vi "Mindsensors Relay Driver Config.vi"(10 "Node Data":T3, 11 "NXT":T1) -> ()   [LabVIEW 2010]
uses:
  <vilib>/NXT/Subs/LVHSConnector.ctl
  Datatypes/Node.ctl
  UI Controls/PlugInControls/Pluginbackground.ctl
  <vilib>/NXT/Subs/MotorOutput.ctl
  <vilib>/Utility/miscctls.llb/LVPointTypeDef.ctl
  ConvertNodeAddrLEGOMotor.vi
  <vilib>/NXT/Dual Mode Library/Motors/MotorBrake.vi
  <vilib>/NXT/Dual Mode Library/Motors/MotorOn.vi
  <vilib>/NXT/Dual Mode Library/Motors/MotorReverse.vi
  <vilib>/NXT/Dual Mode Library/Motors/MotorCoast.vi
  ConvertNodeAddrSensor.vi
panel:
  in  "NXT 2":T1
  out "Output Port":T2=3 items=["Port A"=0, "Port B"=1, "Port C"=2, "Ports A & B"=4, "Ports A & C"=5, "Ports B & C"=6, "All Ports"=3]
  out "String":string
  in  "Relay":u16(ring) items=["Off", "Relay 1", "Relay 2"]
  in  "Device Address":string
  in  "NXT Port":string
  in  "Name":string
  out "Headline":string="Type (auto populated)"
  in  "Sensor Parameters":string
  in  "Instance Specific Data":cluster{"Example Data":dbl, "Numeric":dbl}
  in  "Reset":bool
  in  "Save":bool
  in  "Stop":bool
  out "Background":T4=TRUE
  # "<- No controls below this line"
  # "Common controls such as Buttons, Rings, Sliders, Graphs, Decorations, etc can be found in the <labview>\\Targets\\NI\\NXT\\NXT Toolkit\\Schematic Editor\\UI Controls\\Plugin Controls\\ folder. Use these controls when possible to ensure a consistent look and feel with LabVIEW Education Edition."
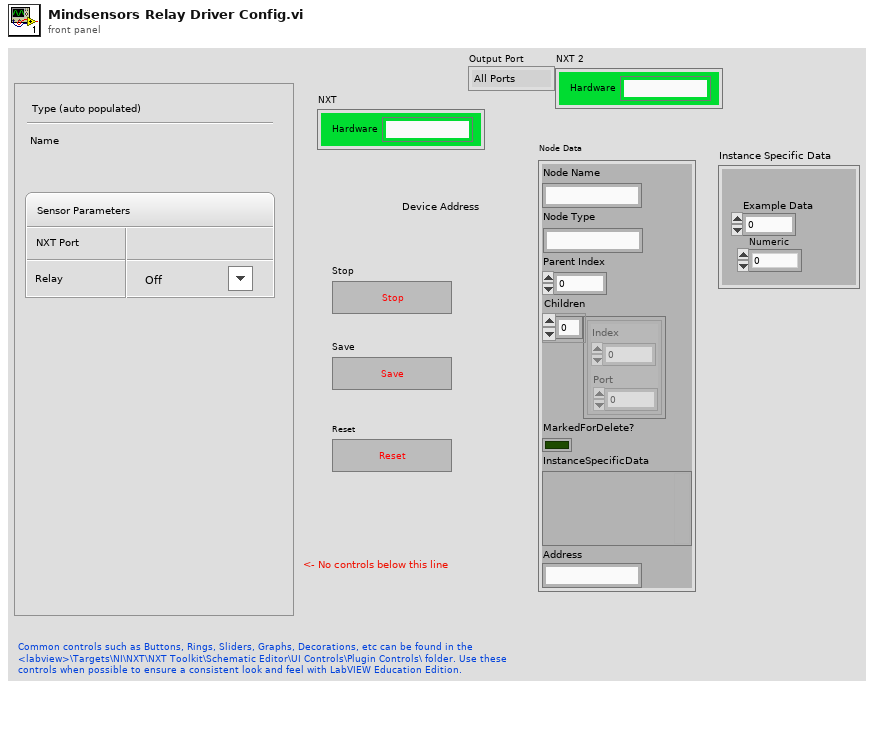
[diagram p1: front panel]
types:
  T1 = typedef "LVHSConnector.ctl" = cluster{"Hardware":string, "Flattened String":string}
  T2 = typedef "MotorOutput.ctl" = u8
  T3 = typedef "Node.ctl" = cluster{"Node Name":string, "Node Type":string, "Parent Index":i16, "Children":cluster{"Index":u16, "Port":u16}[], "MarkedForDelete?":bool, "InstanceSpecificData":variant, "Address":string}
  T4 = typedef "Pluginbackground.ctl" = bool
  T5 = typedef "LVPointTypeDef.ctl" = cluster{"Horizontal":i16, "Vertical":i16}
  T6 = enum8{"Enabled", "Disabled", "Disabled and Grayed Out"}
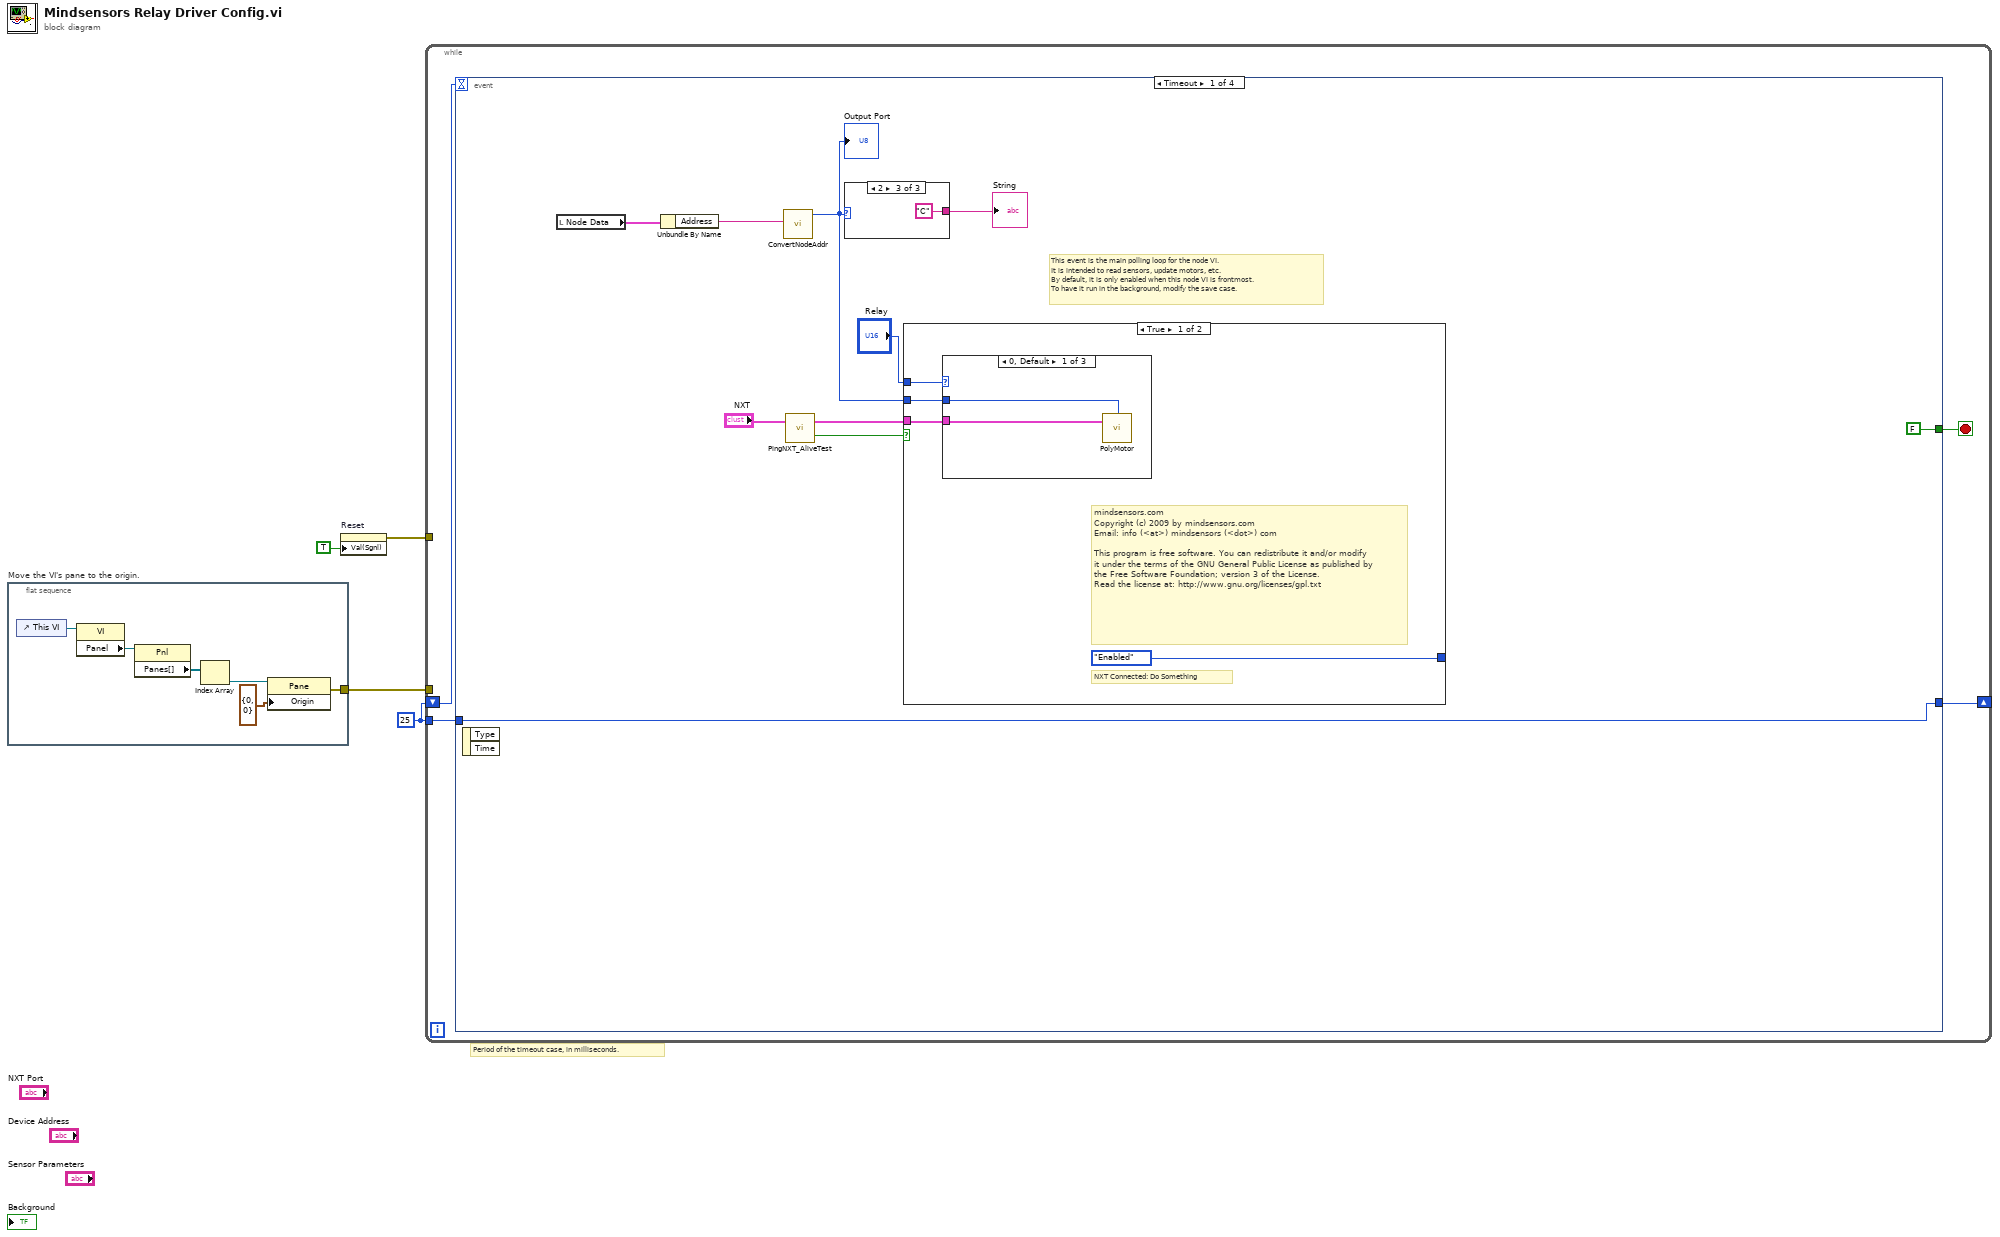
[diagram p0: block diagram]
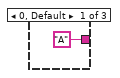
[diagram p2: hidden frame]
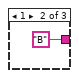
[diagram p3: hidden frame]
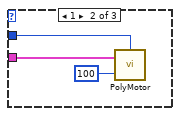
[diagram p4: hidden frame]
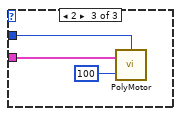
[diagram p5: hidden frame]
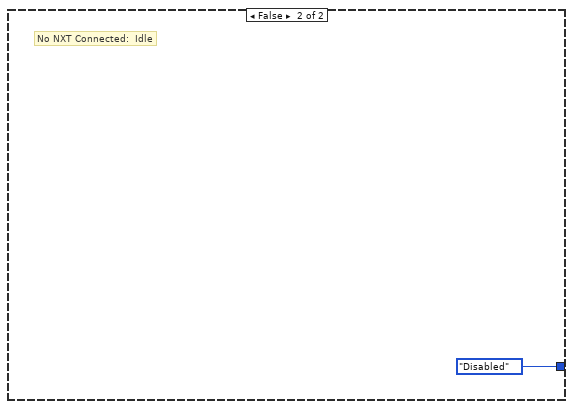
[diagram p6: hidden frame]
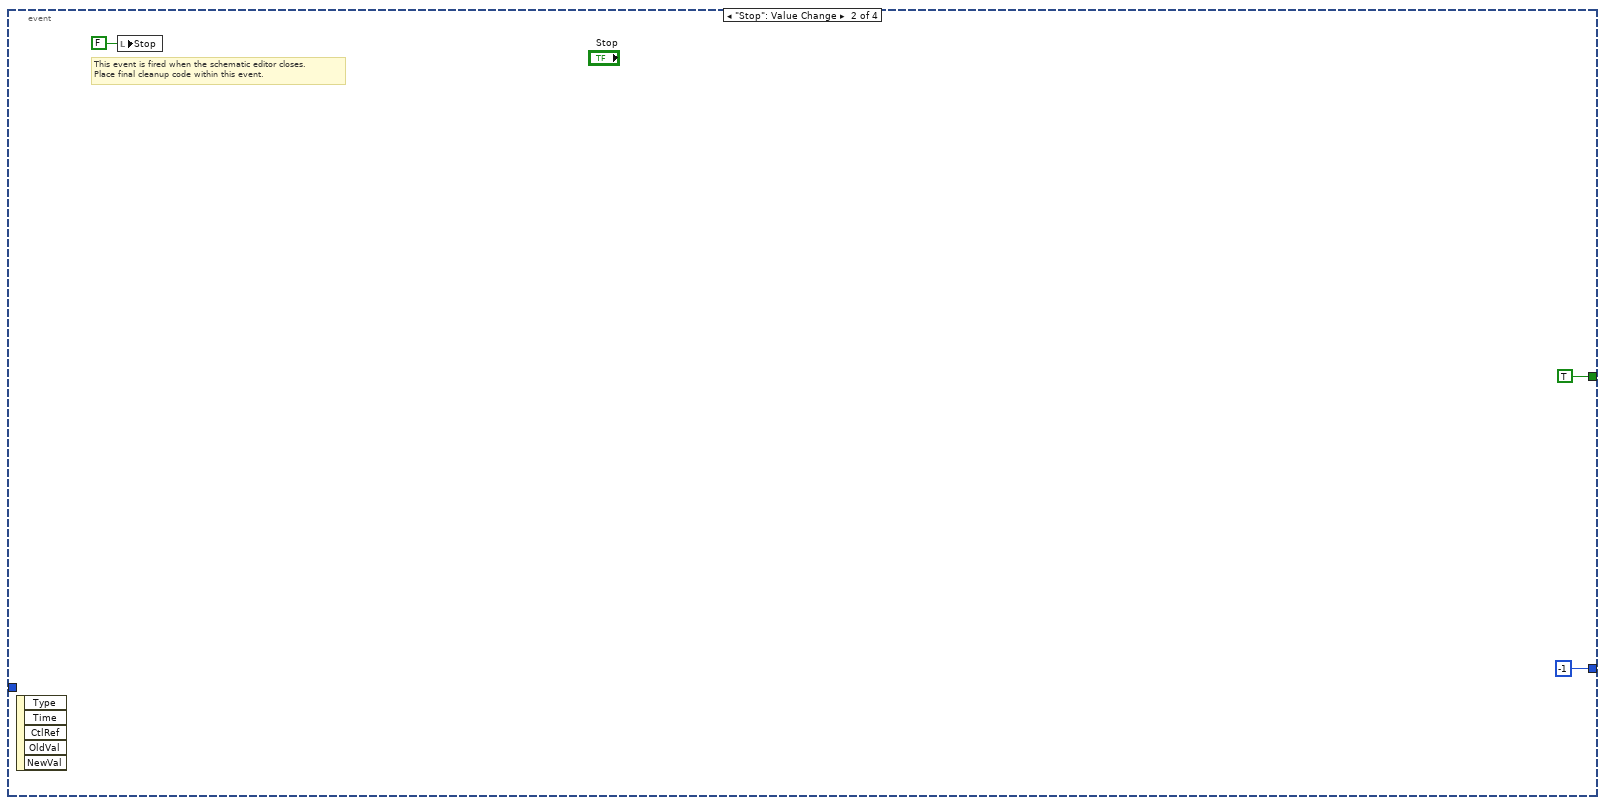
[diagram p7: hidden frame]
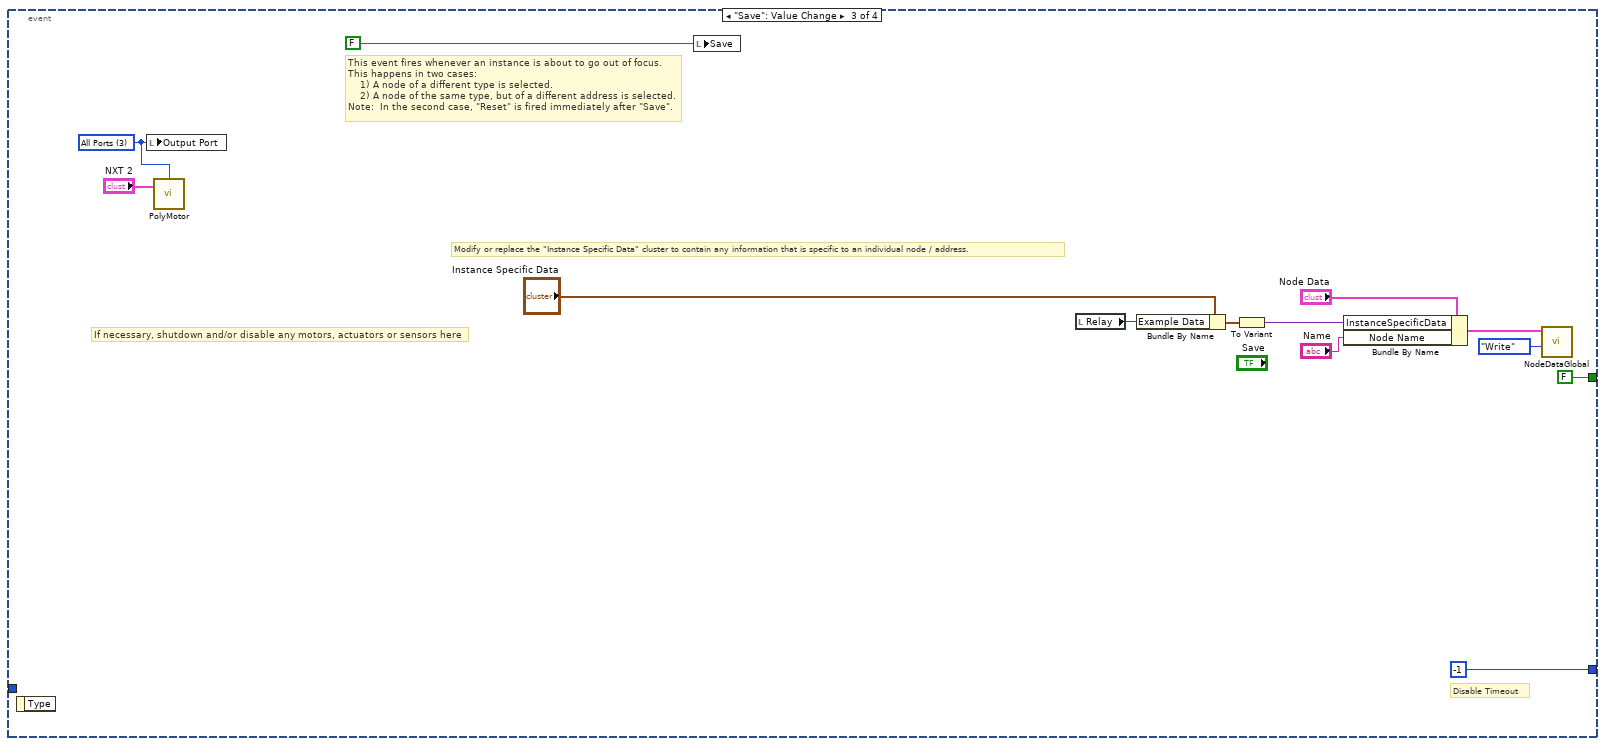
[diagram p8: hidden frame]
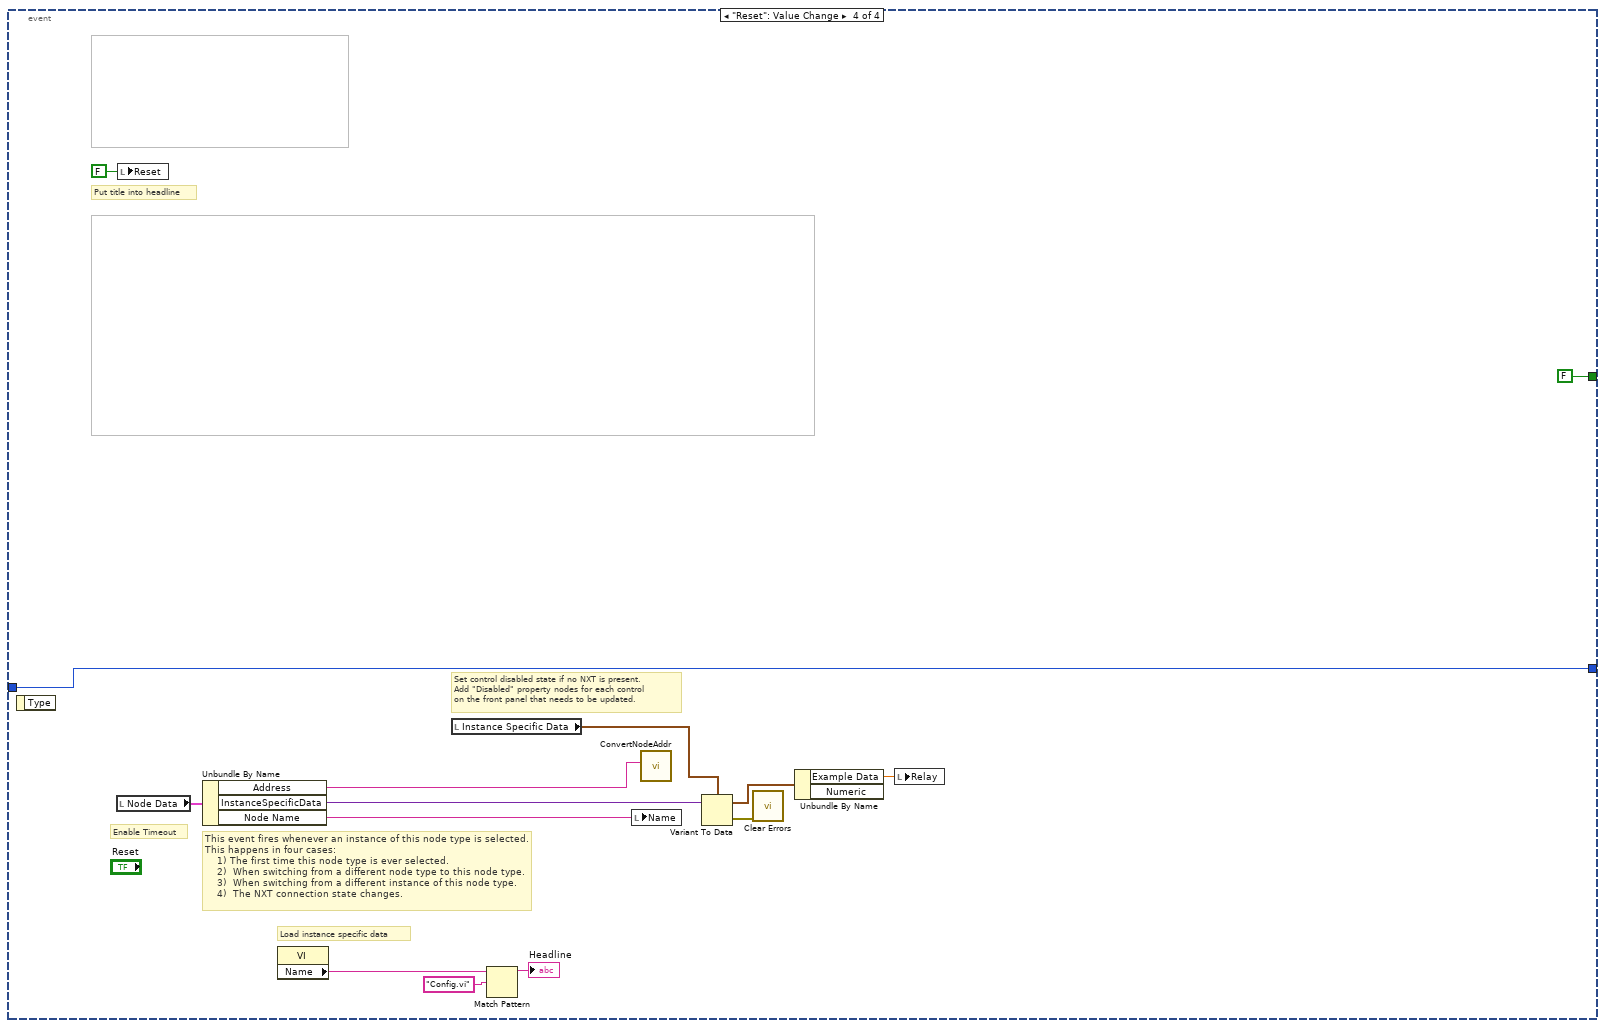
[diagram p9: hidden frame]
diagram:
  w2 = 25
  # "Period of the timeout case, in milliseconds."
  n1 = flat-sequence "Move the VI's pane to the origin." {
    tunnel: [w5] -> w1
    frame #0 {
      n2 = control-ref of="This VI"() -> (w6:refnum<vi>)
      n3 = property class="VI"(reference=w6) -> ("Panel"=w7:refnum<vi>)  [unwired: 1 in, 2 out]
      n4 = property class="Pnl"(reference=w7) -> ("Panes[]"=w8:refnum<vi>[])  [unwired: 1 in, 2 out]
      n5 = Index Array(array=w8) -> (element=w9:refnum<vi>)  [unwired: 1 in]
      n6 = property class="Pane"(reference=w9, "Origin"=T5 {"Horizontal"=0, "Vertical"=0}) -> (error out=w5:errorcluster)  [unwired: 1 in, 1 out]
    }
  }
  n7 = property on="Reset" class="Bool (strict)"("Val(Sgnl)"=TRUE ("Value (Signaling)")) -> (error out=w3:errorcluster)  [unwired: 2 in, 1 out]
  n8 = while {
    tunnel: w3 -> [_]
    shift-right: [w12] -> _
    shift-left: w2 -> [w13]
    tunnel: w2 -> [w11]
    tunnel: w1 -> [_]
    stop <- w14 stop-if-true
    n9 = event shown="[0] Timeout" {
      selector: _ -> [_ _ _ _]
      dyn-events: _ -> [_ _ _ _]
      timeout: w13 -> [_ _ _ _]
      tunnel: [FALSE TRUE FALSE FALSE] -> w14
      tunnel: [w23 -1 -1 w66] -> w12
      tunnel: w11 -> [w23 _ _ w66]
      event Timeout {
        # "This event is the main polling loop for the node VI.\nIt is intended to read sensors, update motors, etc.\nBy default, it is only enabled when this node VI is frontmost.\nTo have it run in the background, modify the save case."
        n10 = event-data() -> ()  [unwired: 1 in, 2 out]
        n11 = local read "Node Data"() -> (w21:T3)
        n12 = Unbundle By Name(w21) -> ("Address"=w18:string)
        n13 = call-poly "ConvertNodeAddr.vi"("Motor Port"=w18) -> ("Output Port"=w16:T2)  [unwired: 8 in, 2 out]
        "Output Port" <- w16
        n14 = call <vilib>:"PingNXT_AliveTest.vi"("NXT"="NXT") -> ("connected?"=w20:bool, "NXT"=w19:T1)  [unwired: 1 in]
        n15 = case shown="2" w16 {
          tunnel: ["A" ("String") "B" ("String") "C" ("String")] -> w15
          frame 0, Default {
          }
          frame 1 {
          }
          frame 2 {
          }
        }
        "String" <- w15
        n16 = case shown="True" w20 {
          tunnel: [T6."Enabled" ("Disabled") T6."Disabled" ("Disabled")] -> _
          tunnel: w19 -> [w30 _]
          tunnel: "Relay" -> [w29 _]
          tunnel: w16 -> [w28 _]
          frame True {
            # "mindsensors.com\nCopyright (c) 2009 by mindsensors.com\nEmail: info (<at>) mindsensors (<dot>) com\n\nThis program is free software. You can redistribute it and/or modify\nit under the terms of the GNU General Public License as published by\nthe Free Software Foundation; version 3 of the License.\nRead the license at: http://www.gnu.org/licenses/gpl.txt"
            # "NXT Connected: Do Something"
            n17 = case shown="0, Default" w29 {
              tunnel: w30 -> [w33 w35 w39]
              tunnel: w28 -> [w32 w34 w37]
              frame 0, Default {
                n18 = call-poly <vilib>:"PolyMotor.vi"("NXT"=w33, "Port (All Ports)"=w32) -> ()  [unwired: 2 in, 1 out]
              }
              frame 1 {
                n19 = call-poly <vilib>:"PolyMotor.vi"("Power (75)"=100, "NXT"=w35, "Output Port (All Ports)"=w34) -> ()  [unwired: 1 in, 1 out]
              }
              frame 2 {
                n20 = call-poly <vilib>:"PolyMotor.vi"("Power (75)"=100, "NXT"=w39, "Output Port (All Ports)"=w37) -> ()  [unwired: 1 in, 1 out]
              }
            }
          }
          frame False {
            # "No NXT Connected:  Idle"
          }
        }
      }
      event "Stop": Value Change {
        # "This event is fired when the schematic editor closes.\nPlace final cleanup code within this event."
        n21 = event-data() -> ()  [unwired: 1 in, 5 out]
        n22 = local write "Stop"(FALSE ("stop")) -> ()
      }
      event "Save": Value Change {
        w45 = T2 3 items=["Port A", "Port B", "Port C", "All Ports"] ("Output Port")
        # "If necessary, shutdown and/or disable any motors, actuators or sensors here"
        # "Modify or replace the \"Instance Specific Data\" cluster to contain any information that is specific to an individual node / address."
        # "Disable Timeout"
        # "This event fires whenever an instance is about to go out of focus.\nThis happens in two cases:\n    1) A node of a different type is selected.\n    2) A node of the same type, but of a different address is selected.\nNote:  In the second case, \"Reset\" is fired immediately after \"Save\"."
        n23 = event-data() -> ()  [unwired: 1 in, 1 out]
        n24 = local write "Output Port"(w45) -> ()
        n25 = call-poly <vilib>:"PolyMotor.vi"("NXT"="NXT 2", "Port (All Ports)"=w45) -> ()  [unwired: 2 in, 1 out]
        n26 = local write "Save"(FALSE ("stop")) -> ()
        n27 = local read "Relay"() -> (w46:u16)
        n28 = Bundle By Name(cluster="Instance Specific Data", "Example Data"=w46) -> (w47:cluster{"Example Data":dbl, "Numeric":dbl})
        n29 = To Variant(anything=w47) -> (Variant=w54:variant)
        n30 = Bundle By Name(cluster="Node Data", "InstanceSpecificData"=w54, "Node Name"="Name") -> (w53:T3)
        n31 = call "NodeDataGlobal.vi"("Action"=enum16{"Read", "Write"}."Write", "Node Data In"=w53) -> ()  [unwired: 8 in, 2 out]
      }
      event "Reset": Value Change {
        # "Set control disabled state if no NXT is present.\nAdd \"Disabled\" property nodes for each control\non the front panel that needs to be updated."
        # "Load instance specific data"
        # "Enable Timeout"
        # "This event fires whenever an instance of this node type is selected.\nThis happens in four cases:\n    1) The first time this node type is ever selected.\n    2)  When switching from a different node type to this node type.\n    3)  When switching from a different instance of this node type. \n    4)  The NXT connection state changes."
        # "Put title into headline"
        n32 = event-data() -> ()  [unwired: 1 in, 1 out]
        n33 = local read "Node Data"() -> (w67:T3)
        n34 = local write "Reset"(FALSE ("Reset")) -> ()
        n35 = Unbundle By Name(w67) -> ("Address"=w58:string, "InstanceSpecificData"=w68:variant, "Node Name"=w60:string)
        n36 = property class="VI"() -> ("Name"=w62:string)  [unwired: 2 in, 2 out]
        n37 = local read "Instance Specific Data"() -> (w65:cluster{"Example Data":dbl, "Numeric":dbl})
        n38 = Match Pattern(string=w62, regular expression="Config.vi") -> (before substring=→"Headline":string)  [unwired: 1 in, 3 out]
        n39 = local write "Name"(w60) -> ()
        n40 = call-poly "ConvertNodeAddr.vi"("Sensor Port"=w58) -> ()  [unwired: 6 in, 5 out]
        n41 = Variant To Data(Variant=w68, type=w65) -> (error out=w64:errorcluster, data=w59:cluster{"Example Data":dbl, "Numeric":dbl})  [unwired: 1 in]
        n42 = call <vilib>:"Clear Errors.vi"("error in (no error)"=w64) -> ()  [unwired: 6 in, 1 out]
        n43 = Unbundle By Name(w59) -> ("Example Data"=w57:dbl)  [unwired: 1 out]
        n44 = local write "Relay"(w57) -> ()
      }
    }
  }
